vi "Close Joysticks.vi"(8 "error in":errorcluster) -> (0 "error out":errorcluster)   [LabVIEW 2018]
uses:
  TypeDefs/typedef_enum_Refnums.ctl
  <vilib>/Rock Robotics/WPI/Utilities/WPI_GetSetVariantRefNum.vi
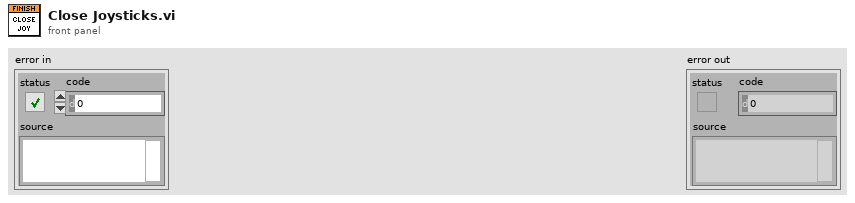
[diagram p1: front panel]
types:
  T1 = typedef "typedef_enum_Refnums.ctl" = enum16{"Ball_Encoder", "Ball_Motor", "Camera", "Linefollow_3", "Linefollow_2", "Linefollow_1", "Gyro", "Hatch_Solenoid", "Climb_Back_Solenoid", "Arm_Encoder", "Arm_Motor", "Lift_Encoder", "Drive", "Drive_Motor_R", "Drive_Motor_L", "Drive_Encoder_R", "Drive_Encoder_L", "Joy_R", "Joy_L", "Wrist_Motor", "Wrist_Encoder", "Climb Upper Limit", "Climb Lower Limit ", "Climb_Front_Motor"}
  T2 = typedef "WPI_JoystickDevRef.ctl" = cluster{"Device":T3}
  T3 = typedef "WPI_JoystickDeviceEnum.ctl" = enum16{"USB 0", "USB 1", "USB 2", "USB 3", "USB 4", "USB 5"}
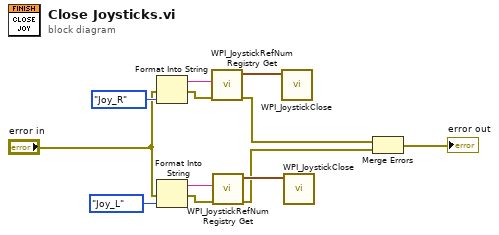
[diagram p0: block diagram]
diagram:
  n1 = Format Into String(error in="error in", typedef_enum_Refnums."Joy_R" ("RefNums")) -> (resulting string=w8:string, error out=w6:errorcluster)  [unwired: 2 in]
  n2 = Format Into String(error in="error in", typedef_enum_Refnums."Joy_L" ("RefNums")) -> (resulting string=w9:string, error out=w3:errorcluster)  [unwired: 2 in]
  n3 = call <vilib>:"WPI_JoystickRefNum Registry Get.vi"("error in (no error)"=w6, "refnum name"=w8) -> ("error out"=w5:errorcluster, "JoystickDevRef"=w12:T2)  [unwired: 8 in]
  n4 = call <vilib>:"WPI_JoystickRefNum Registry Get.vi"("error in (no error)"=w3, "refnum name"=w9) -> ("error out"=w2:errorcluster, "JoystickDevRef"=w11:T2)  [unwired: 8 in]
  n5 = call <vilib>:"WPI_JoystickClose.vi"("JoystickDevRef"=w12) -> ()  [unwired: 11 in]
  n6 = call <vilib>:"WPI_JoystickClose.vi"("JoystickDevRef"=w11) -> ()  [unwired: 11 in]
  n7 = Merge Errors(w5, w2) -> (→"error out":errorcluster)
